vi "ECGGen-Waveform.vi"(11 "Sampling Rate (Hz)":dbl=10000.0) -> (2 "ECG Waveform":dbl[](array[numeric]))   [LabVIEW 2015]
uses:
  <vilib>/Analysis/NI_AALBase.lvlib
  <vilib>/Analysis/3filter.llb/Butterworth Filter (DBL).vi
  <vilib>/Analysis/3filter.llb/Filter Passband Type.ctl
panel:
  in  "Duration (s)":dbl=2.0
  out "Waveform Graph":dbl[](graph)
  in  "Noise (uV)":dbl=50.0
  in  "Jitter (%)":dbl=2.5
  in  "HR (bpm)":dbl=250.0
  out "error out":errorcluster
  in  "error in (no error)":errorcluster
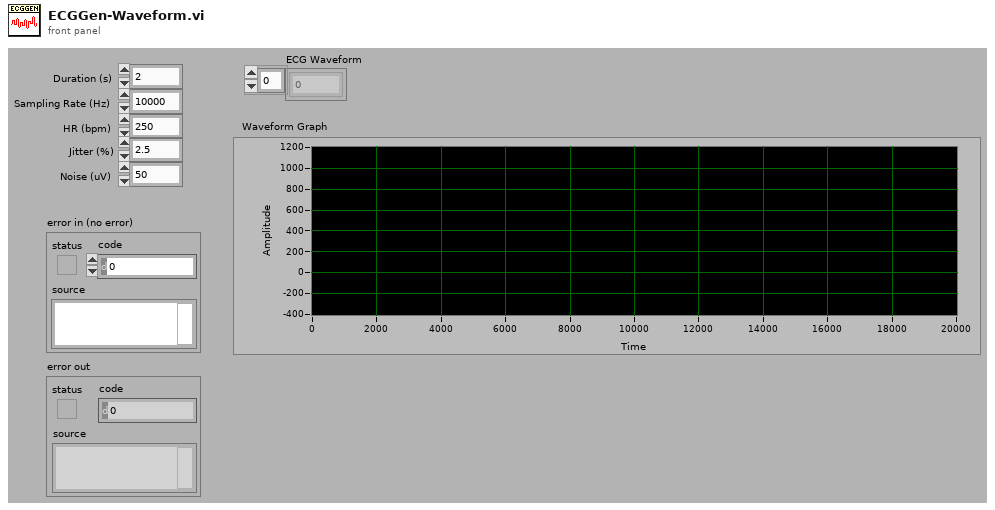
[diagram p1: front panel]
types:
  T1 = typedef "NI_AALBase.lvlib/Filter Passband Type.ctl" = enum32{"Lowpass", "Highpass", "Bandpass", "Bandstop"}
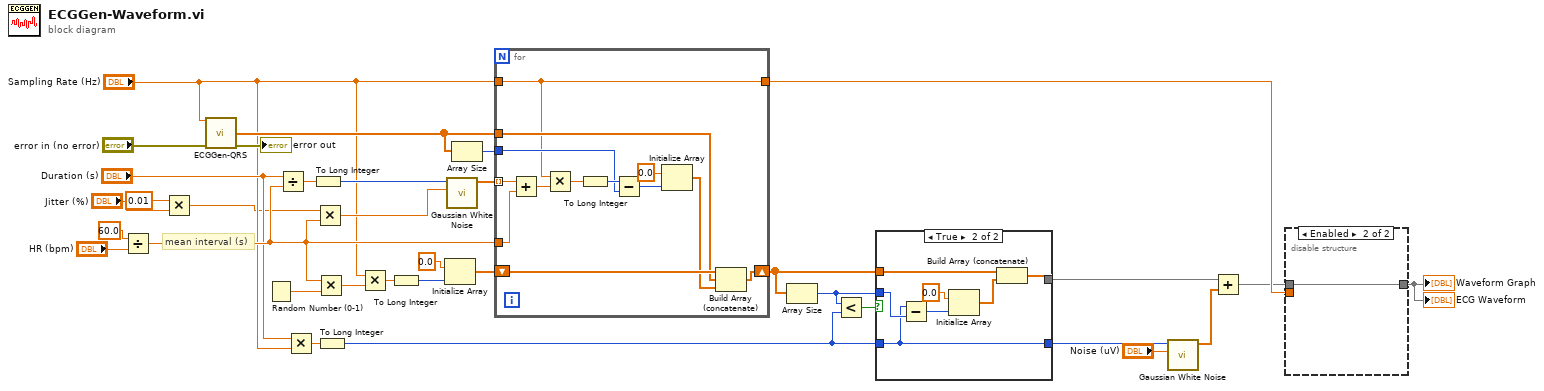
[diagram p0: block diagram]
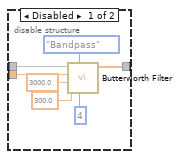
[diagram p2: hidden frame]
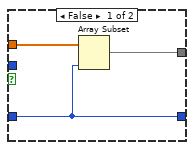
[diagram p3: hidden frame]
diagram:
  # "mean interval (s)"
  n1 = Divide(x=60.0, y="HR (bpm)") -> (x/y=w19:dbl)
  n2 = Multiply(x=0.01, y="Jitter (%)") -> (x*y=w5:dbl)
  n3 = call "ECGGen-QRS.vi"("Sample Rate (Hz)"="Sampling Rate (Hz)", "error in (no error)"="error in (no error)") -> ("One ECG"=w21:dbl[], "error out"=→"error out":errorcluster)  [unwired: 12 in]
  n4 = Random Number (0-1)() -> (number: 0 to 1=w30:dbl)
  n5 = Divide(x="Duration (s)", y=w19) -> (x/y=w31:dbl)
  n6 = Multiply(x="Duration (s)", y="Sampling Rate (Hz)") -> (x*y=w17:dbl)
  n7 = To Long Integer(number=w31) -> (32bit integer=w28:i32)
  n8 = Multiply(x=w5, y=w19) -> (x*y=w27:dbl)
  n9 = Multiply(x=w19, y=w30) -> (x*y=w25:dbl)
  n10 = To Long Integer(number=w17) -> (32bit integer=w11:i32)
  n11 = Multiply(x="Sampling Rate (Hz)", y=w25) -> (x*y=w24:dbl)
  n12 = To Long Integer(number=w24) -> (32bit integer=w23:i32)
  n13 = Initialize Array(0.0 ("element"), w23) -> (w22:dbl[])
  n14 = call <vilib>:"Gaussian White Noise.vi"("standard deviation"=w27, "samples"=w28) -> ("Gaussian noise pattern"=w26:dbl[])  [unwired: 8 in, 1 out]
  n15 = Array Size(array=w21) -> (size(s)=w20:i32)
  n16 = for {
    tunnel: w26 -> [w45] mode=indexing
    shift-right: [w46] -> w12
    shift-left: w22 -> [w47]
    tunnel: w21 -> [w43]
    tunnel: w20 -> [w40]
    tunnel: "Sampling Rate (Hz)" -> [w35]
    tunnel: w19 -> [w36]
    tunnel: [w35] -> w3
    n17 = Add(x=w45, y=w36) -> (x+y=w37:dbl)
    n18 = Multiply(x=w35, y=w37) -> (x*y=w44:dbl)
    n19 = To Long Integer(number=w44) -> (32bit integer=w41:i32)
    n20 = Subtract(x=w41, y=w40) -> (x-y=w39:i32)
    n21 = Initialize Array(0.0 ("element"), w39) -> (w38:dbl[])
    n22 = Build Array (concatenate)(w47, w43, w38) -> (w46:dbl[])
  }
  n23 = Array Size(array=w12) -> (size(s)=w9:i32)
  n24 = Less?(x=w9, y=w11) -> (x < y?=w13:bool)
  n25 = case shown="True" w13 {
    tunnel: w12 -> [w50 w57]
    tunnel: w11 -> [w48 w51]
    tunnel: [w49 w56] -> w10
    tunnel: w9 -> [_ w52]
    tunnel: [w48 w51] -> w8
    frame False {
      n26 = Array Subset(array=w50, length=w48) -> (w49:dbl[])  [unwired: 1 in]
    }
    frame True {
      n27 = Subtract(x=w51, y=w52) -> (x-y=w53:i32)
      n28 = Initialize Array(0.0 ("element"), w53) -> (w54:dbl[])
      n29 = Build Array (concatenate)(w57, w54) -> (w56:dbl[])
    }
  }
  n30 = call <vilib>:"Gaussian White Noise.vi"("standard deviation"="Noise (uV)", "samples"=w8) -> ("Gaussian noise pattern"=w6:dbl[])  [unwired: 8 in, 1 out]
  n31 = Add(x=w10, y=w6) -> (x+y=w2:dbl[])
  n32 = disable-structure shown="Enabled" {
    disable-tunnel: w3 -> [w60 _]
    disable-tunnel: w2 -> [w59 w65]
    disable-tunnel: [w58 w65] -> w1
    frame Disabled {
      n33 = call-poly <vilib>:"Butterworth Filter.vi"("order"=4, "filter type"=Filter_Passband_Type."Bandpass", "low cutoff freq: fl"=300.0, "high cutoff freq: fh"=3000.0, "sampling freq: fs"=w60, "X"=w59) -> ("Filtered X"=w58:dbl[])  [unwired: 2 in, 1 out]
    }
    frame Enabled {
    }
  }
  "Waveform Graph" <- w1
  "ECG Waveform" <- w1
